vi "Update State Value Table Change Controls.vi"(6 "update all controls?":bool, 7 "Routing Channel Page Controls":T2, 8 "error in":errorcluster, 9 "old modified state and value":T1, 10 "new modified state and value":T1, 11 "all states and values":T1[](array[typedef])) -> (0 "error out":errorcluster)   [LabVIEW 2020, in "Routing and Faulting System Explorer.lvlib"]
uses:
  Routing and Faulting System Explorer.lvlib
  Routing Channel Page Controls.ctl
  State-Value Row.ctl
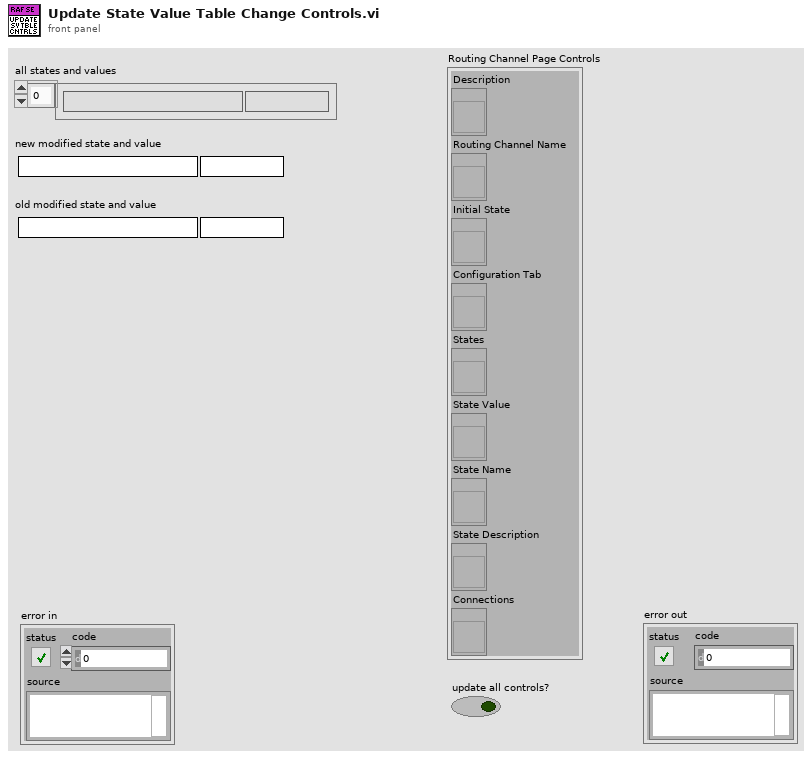
[diagram p1: front panel]
types:
  T1 = typedef "Routing and Faulting System Explorer.lvlib/State-Value Row.ctl" = cluster{"State":string, "State Value":string}
  T2 = typedef "Routing and Faulting System Explorer.lvlib/Routing Channel Page Controls.ctl" = cluster{"Description":refnum<vi>, "Routing Channel Name":refnum<vi>, "Initial State":refnum<vi>, "Configuration Tab":refnum<vi>, "States":refnum<vi>, "State Value":refnum<vi>, "State Name":refnum<vi>, "State Description":refnum<vi>, "Connections":refnum<vi>}
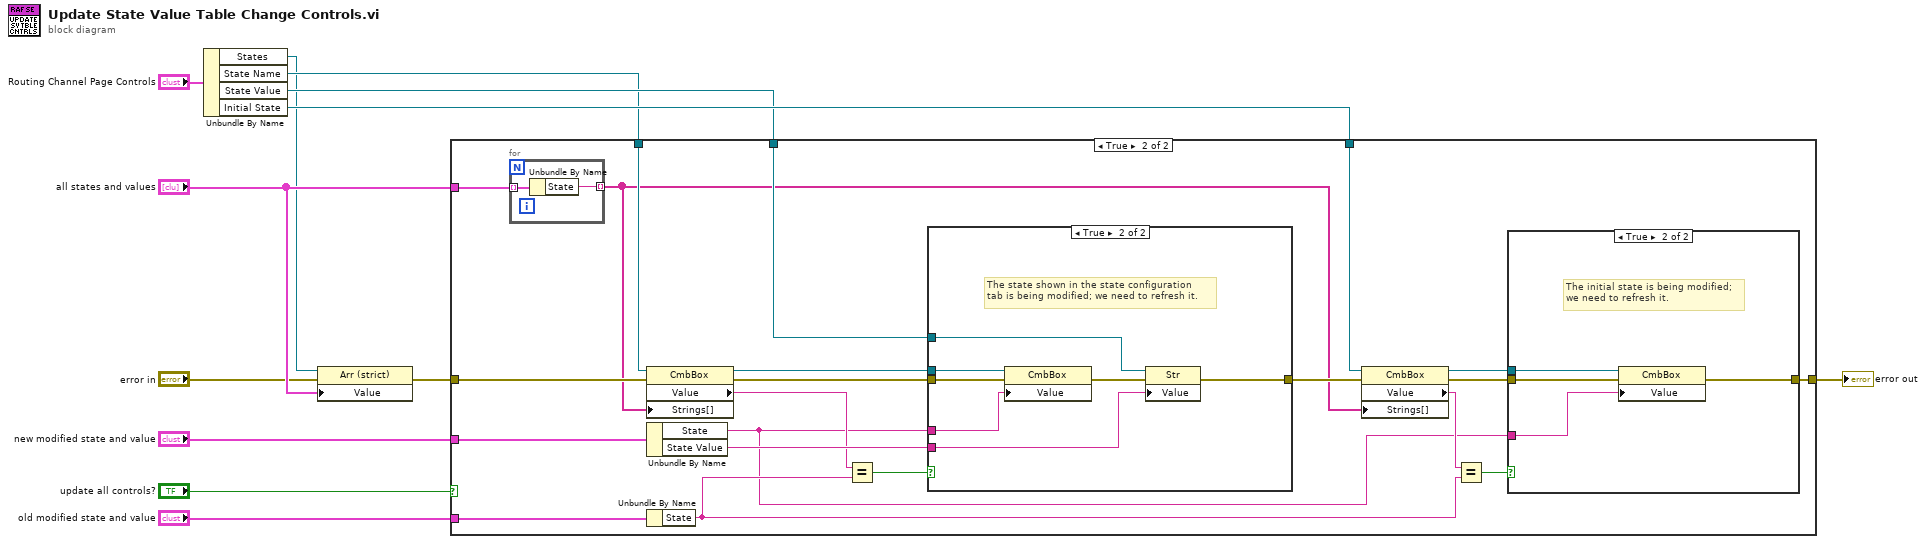
[diagram p0: block diagram]
diagram:
  n1 = Unbundle By Name("Routing Channel Page Controls") -> ("States"=w3:refnum<vi>, "State Name"=w5:refnum<vi>, "State Value"=w9:refnum<vi>, "Initial State"=w12:refnum<vi>)
  n2 = property class="Arr (strict)"(reference=w3, error in="error in", "Value"="all states and values") -> (error out=w10:errorcluster)  [unwired: 1 out]
  n3 = case shown="True" "update all controls?" {
    tunnel: [w13 w18] -> w4
    tunnel: w5 -> [_ w26]
    tunnel: "old modified state and value" -> [_ w33]
    tunnel: "new modified state and value" -> [_ w32]
    tunnel: w9 -> [_ w27]
    tunnel: w10 -> [w13 w31]
    tunnel: "all states and values" -> [_ w30]
    tunnel: w12 -> [_ w24]
    frame False {
    }
    frame True {
      n4 = for {
        tunnel: w30 -> [w44] mode=indexing
        tunnel: [w43] -> w22 mode=indexing
        n5 = Unbundle By Name(w44) -> ("State"=w43:string)
      }
      n6 = property class="CmbBox"(reference=w26, error in=w31, "Strings[]"=w22) -> (reference out=w14:refnum<vi>, error out=w29:errorcluster, "Value"=w21:string)
      n7 = Unbundle By Name(w32) -> ("State"=w16:string, "State Value"=w25:string)
      n8 = Unbundle By Name(w33) -> ("State"=w20:string)
      n9 = Equal?(x=w21, y=w20) -> (x = y?=w28:bool)
      n10 = case shown="True" w28 {
        tunnel: [w35 w42] -> w34
        tunnel: w29 -> [w35 w41]
        tunnel: w27 -> [_ w40]
        tunnel: w16 -> [_ w38]
        tunnel: w25 -> [_ w37]
        tunnel: w14 -> [_ w36]
        frame False {
        }
        frame True {
          # "The state shown in the state configuration\ntab is being modified; we need to refresh it."
          n11 = property class="CmbBox"(reference=w36, error in=w41, "Value"=w38) -> (error out=w39:errorcluster)  [unwired: 1 out]
          n12 = property class="Str"(reference=w40, error in=w39, "Value"=w37) -> (error out=w42:errorcluster)  [unwired: 1 out]
        }
      }
      n13 = property class="CmbBox"(reference=w24, error in=w34, "Strings[]"=w22) -> (reference out=w15:refnum<vi>, error out=w19:errorcluster, "Value"=w23:string)
      n14 = Equal?(x=w23, y=w20) -> (x = y?=w17:bool)
      n15 = case shown="True" w17 {
        tunnel: w19 -> [w45 w49]
        tunnel: [w45 w48] -> w18
        tunnel: w16 -> [_ w47]
        tunnel: w15 -> [_ w46]
        frame False {
        }
        frame True {
          # "The initial state is being modified;\nwe need to refresh it."
          n16 = property class="CmbBox"(reference=w46, error in=w49, "Value"=w47) -> (error out=w48:errorcluster)  [unwired: 1 out]
        }
      }
    }
  }
  "error out" <- w4
